vi "JSON to TOP file.vi"(8 "error in (no error)":errorcluster, 10 "Capabilities JSON In":string) -> (0 "error out":errorcluster, 2 "Topologies out":T1[](array[typedef]))   [LabVIEW 2015, in "SLSC Switch.lvclass"]
uses:
  SLSC Switch.lvclass
  Controls/Topology.ctl
  Controls/JSON.Topology.ctl
  Controls/JSON.InitialState.ctl
  Controls/JSON.ChannelList.ctl
  Controls/JSON.ConnectionList.ctl
  <vilib>/Utility/config.llb/Write Key (String).vi
  <vilib>/Utility/config.llb/NI_LVConfig.lvlib
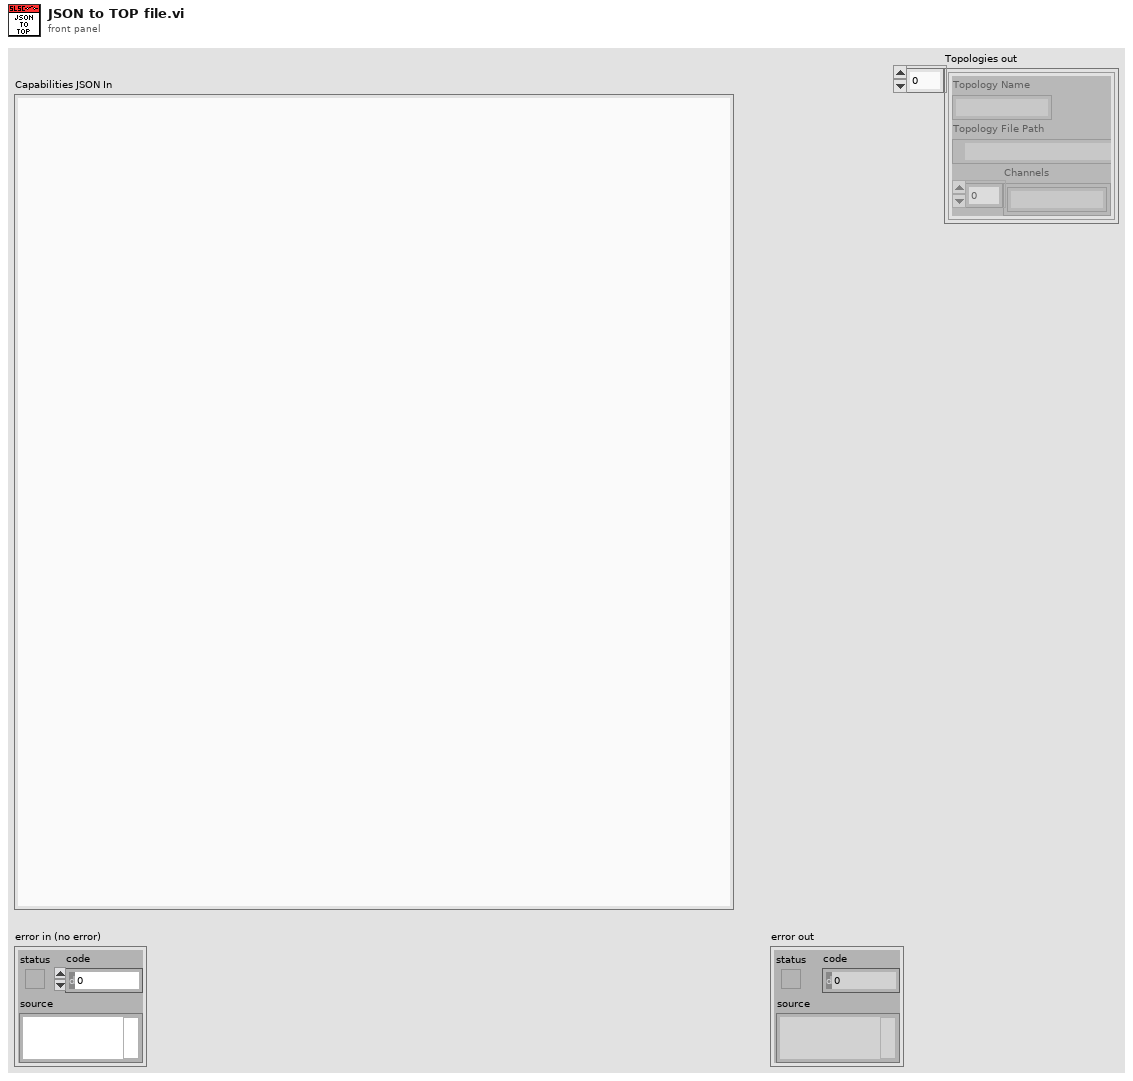
[diagram p1: front panel]
types:
  T1 = typedef "SLSC Switch.lvclass/Topology.ctl" = cluster{"Topology Name":string, "Topology File Path":path, "Channels":string[]}
  T2 = typedef "SLSC Switch.lvclass/JSON.Topology.ctl" = cluster{"name":string, "InitialState":T3, "ChannelList":T4, "ConnectionList":T5[]}
  T3 = typedef "SLSC Switch.lvclass/JSON.InitialState.ctl" = cluster{"Open":string[], "Close":string[]}
  T4 = typedef "SLSC Switch.lvclass/JSON.ChannelList.ctl" = cluster{"Names":string[]}
  T5 = typedef "SLSC Switch.lvclass/JSON.ConnectionList.ctl" = cluster{"Src":string, "Dest":string, "Relays":string[]}
  T6 = typedef "NI_LVConfig.lvlib/Config Data RefNum.ctl" = refnum<k1>
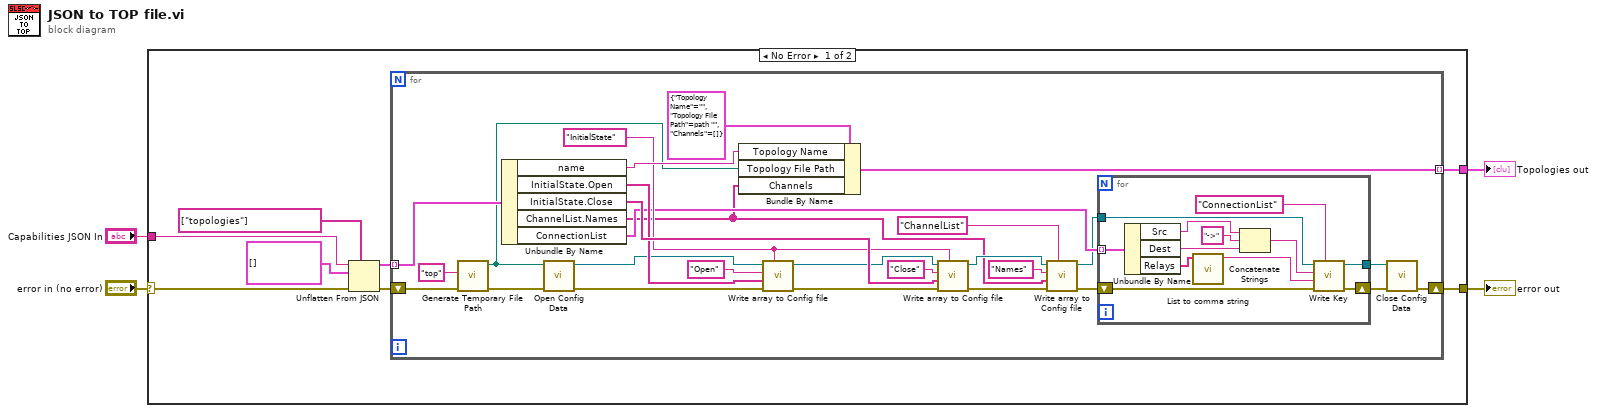
[diagram p0: block diagram]
diagram:
  n1 = case shown="No Error" "error in (no error)" {
    selector: "error in (no error)" -> [w9 w53]
    tunnel: [w5 w53] -> w3
    tunnel: "Capabilities JSON In" -> [w11 _]
    tunnel: [w7 _] -> w1
    frame No Error {
      n2 = Unflatten From JSON(path=string[] ["topologies"], JSON string=w11, type and defaults=T2[] [] ("Array"), error in (no error)=w9) -> (value=w8:T2[], error out=w6:errorcluster)  [unwired: 3 in]
      n3 = for {
        tunnel: w8 -> [w40] mode=indexing
        tunnel: [w34] -> w7 mode=indexing
        shift-right: [w23] -> w5
        shift-left: w6 -> [w25]
        w26 = "InitialState" ("section")
        n4 = call <vilib>:"Generate Temporary File Path.vi"("error in (no error)"=w25, "Temporary File Extension (tmp)"="top") -> ("error out"=w36:errorcluster, "Unique Temporary File Path"=w35:path)  [unwired: 8 in]
        n5 = Unbundle By Name(w40) -> ("name"=w38:string, "InitialState.Open"=w31:string[], "InitialState.Close"=w33:string[], "ChannelList.Names"=w13:string[], "ConnectionList"=w18:T5[])
        n6 = call <vilib>:"Open Config Data.vi"("error in (no error)"=w36, "configuration file path"=w35) -> ("error out"=w29:errorcluster, "refnum"=w24:T6)  [unwired: 7 in, 1 out]
        n7 = Bundle By Name(cluster=T1 {"Topology Name"="", "Topology File Path"=path "", "Channels"=[]} ("Topologies"), "Topology Name"=w38, "Topology File Path"=w35, "Channels"=w13) -> (w34:T1)
        n8 = call "Write array to Config file.vi"("section"=w26, "error in (no error)"=w29, "Array"=w31, "key"="Open", "Refnum in"=w24) -> ("error out"=w28:errorcluster, "refnum out"=w27:T6)  [unwired: 5 in]
        n9 = call "Write array to Config file.vi"("section"=w26, "error in (no error)"=w28, "Array"=w33, "key"="Close", "Refnum in"=w27) -> ("error out"=w21:errorcluster, "refnum out"=w22:T6)  [unwired: 5 in]
        n10 = call "Write array to Config file.vi"("section"="ChannelList", "error in (no error)"=w21, "Array"=w13, "key"="Names", "Refnum in"=w22) -> ("error out"=w16:errorcluster, "refnum out"=w17:T6)  [unwired: 5 in]
        n11 = for {
          tunnel: w18 -> [w52] mode=indexing
          tunnel: w17 -> [w43]
          shift-right: [w44] -> w15
          shift-left: w16 -> [w45]
          tunnel: [w42] -> w14
          n12 = Unbundle By Name(w52) -> ("Src"=w51:string, "Dest"=w49:string, "Relays"=w47:string[])
          n13 = call "List to comma string.vi"("Array"=w47) -> ("String"=w46:string)  [unwired: 10 in]
          n14 = Concatenate Strings(w51, "->" ("string"), w49) -> (w48:string)
          n15 = call-poly <vilib>:"Write Key.vi"("section"="ConnectionList", "error in (no error)"=w45, "value"=w46, "key"=w48, "refnum"=w43) -> ("error out"=w44:errorcluster, "refnum out"=w42:T6)  [unwired: 4 in, 1 out]
        }
        n16 = call <vilib>:"Close Config Data.vi"("error in (no error)"=w15, "refnum"=w14) -> ("error out"=w23:errorcluster)  [unwired: 8 in, 1 out]
      }
    }
    frame Error {
    }
  }
  "error out" <- w3
  "Topologies out" <- w1
